vi "SIFS_ReadPosicAndStat.vi"(0 "VISA resource name":refnum<visa-resource-name>, 2 "ID":string, 3 "FATOR":dbl) -> (1 "Home bit":bool, 4 "Run bit":bool, 5 "VISA Name Out":refnum<visa-resource-name>, 6 "Position":dbl, 7 "Status byte":bool[](array[boolean]), 8 "error out":errorcluster)   [LabVIEW 2018]
panel:
  out "Error":bool
  # "Index"
  # "Moving Error"
  # "Holding Error"
  # "Moving"
  # "I/O#1"
  # "I/O#2"
  # "I/O#3"
  # "Over Temperature"
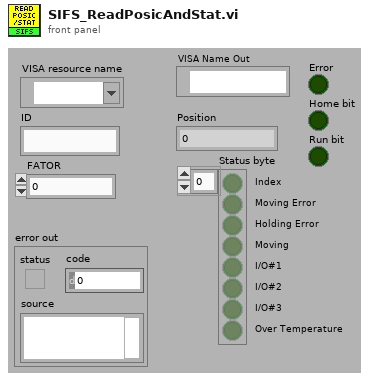
[diagram p1: front panel]
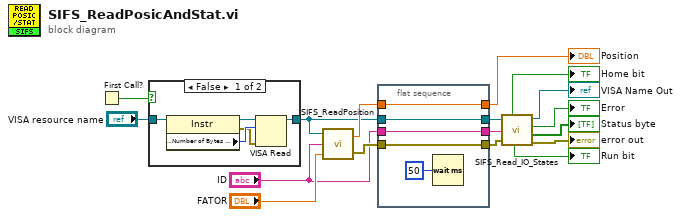
[diagram p0: block diagram]
diagram:
  n1 = First Call?() -> (First Call?: T/F=w15:bool)
  n2 = case shown="False" w15 {
    tunnel: "VISA resource name" -> [w19 w23]
    tunnel: [w18 w23] -> w1
    frame False {
      n3 = property class="Instr"(reference=w19) -> (reference out=w22:refnum<visa-resource-name>, error out=w20:errorcluster, "Serial Settings:Number of Bytes at Serial Port"=w21:u32)  [unwired: 1 in]
      n4 = VISA Read(VISA resource name=w22, byte count=w21, error in (no error)=w20) -> (VISA resource name out=w18:refnum<visa-resource-name>)  [unwired: 3 out]
    }
    frame True {
    }
  }
  n5 = call "SIFS_ReadPosition.vi"("FATOR"="FATOR", "ID"="ID", "VISA resource name"=w1) -> ("error out"=w8:errorcluster, "Position"=w7:dbl)
  n6 = flat-sequence {
    tunnel: w8 -> [w26]
    tunnel: w7 -> [w27]
    tunnel: [w27] -> w6
    tunnel: [w26] -> w5
    tunnel: "ID" -> [w25]
    tunnel: [w25] -> w3
    tunnel: [w24] -> w2
    tunnel: w1 -> [w24]
    frame #0 {
      n7 = Wait (ms)(milliseconds to wait=u32 50) -> ()  [unwired: 1 out]
    }
  }
  n8 = call "SIFS_Read_IO_States.vi"("VISA Name In"=w2, "ID"=w3, "error in"=w5) -> ("Home Bit"=→"Home bit":bool, "Run Bit"=→"Run bit":bool, "VISA Name Out"=→"VISA Name Out":refnum<visa-resource-name>, "Error"=→"Error":bool, "Status Byte"=→"Status byte":bool[], "error out"=→"error out":errorcluster)
  "Position" <- w6
